vi "NI ELVISmx Set Variable Power Supplies.vi"(0 "Device Name":tag="Dev1", 1 "Stop":bool, 2 "Supply+ (V)":dbl min=0.0 max=12.0, 3 "Supply- (V)":dbl min=-12.0 max=0.0, 5 "error in":errorcluster, 7 "Manual +":bool, 8 "Manual -":bool) -> (16 "Manual +?":bool, 17 "Manual -?":bool, 19 "error out":errorcluster)   [LabVIEW 2014]
doc: "This one shot VI sets the voltage of the positive and negative variable voltage supplies on the ELVIS board. The output can be cleared by running the vi again with the Clear button set to true. If this fails power off the NI Elvis Board.\n\nPaul K Dixon\nPhysics 350\nCSUSB Physics"
uses:
  nilvaiu.dll
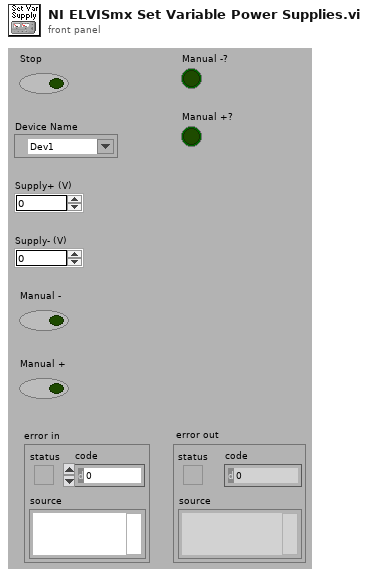
[diagram p1: front panel]
types:
  T1 = typedef "ctl_ProductCategory.ctl" = u16
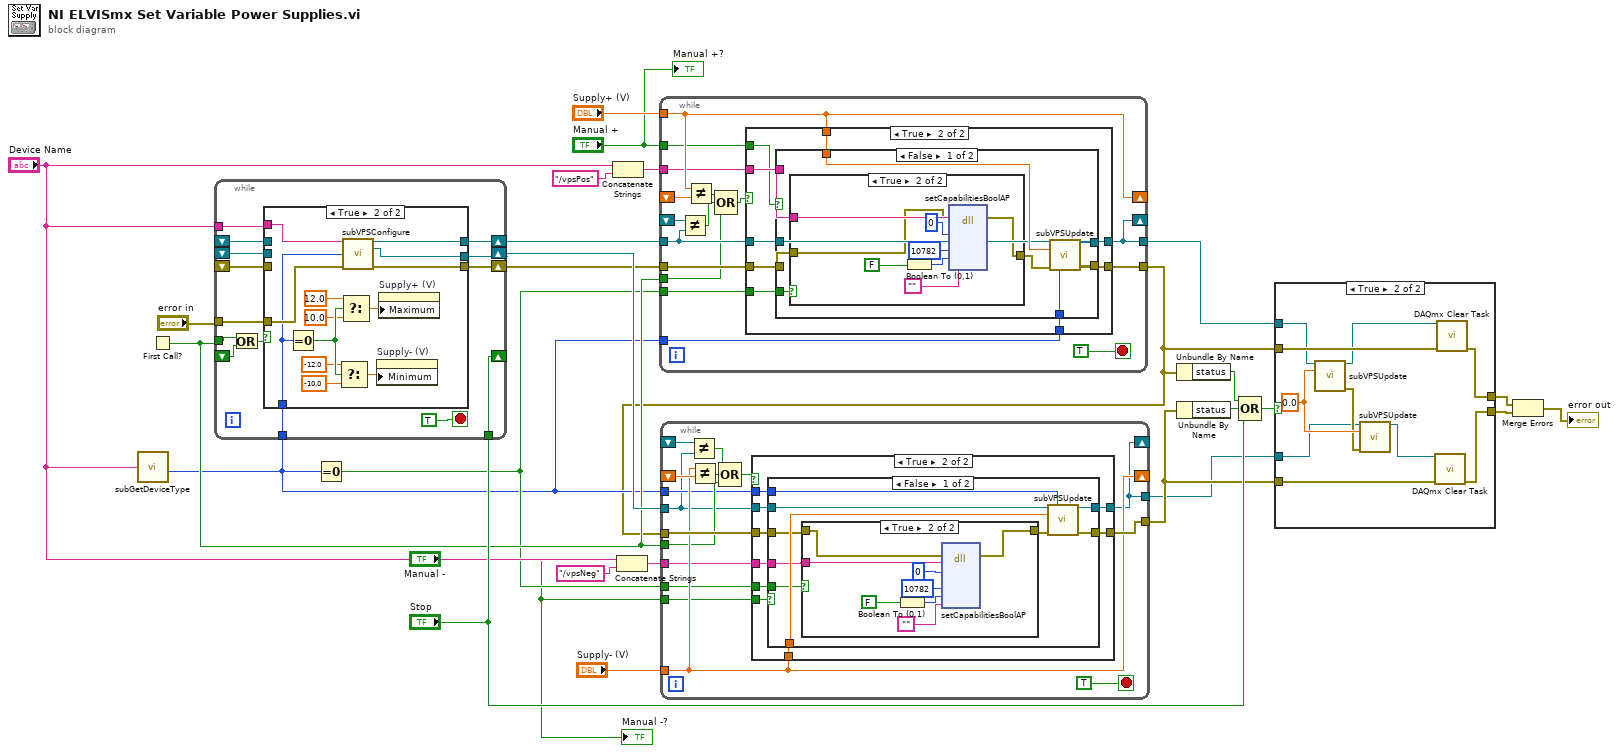
[diagram p0: block diagram]
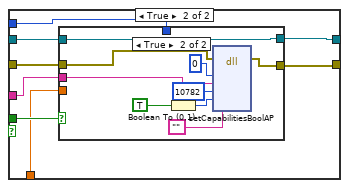
[diagram p4: hidden frame]
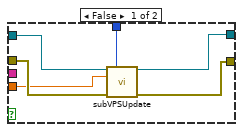
[diagram p5: hidden frame]
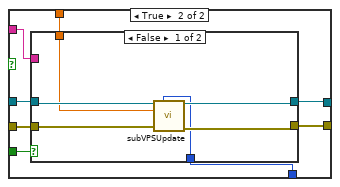
[diagram p8: hidden frame]
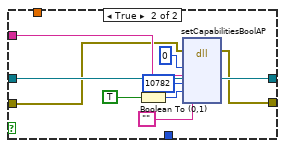
[diagram p9: hidden frame]
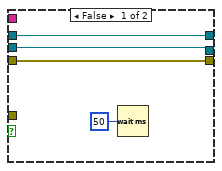
[diagram p11: hidden frame]
diagram:
  n1 = call <vilib>:"subGetDeviceType.vi"("DAQmx Device Name"="Device Name") -> ("Product Category"=w5:T1)  [unwired: 4 out]
  n2 = First Call?() -> (First Call?: T/F=w12:bool)
  n3 = while {
    tunnel: "error in" -> [w41]
    tunnel: w12 -> [w40]
    tunnel: "Device Name" -> [w38]
    tunnel: "Stop" -> [w36]
    shift-right: [w36] -> _
    shift-left: _ -> [w35]
    shift-right: [w34] -> w2
    shift-left: _ -> [w33]
    shift-right: [w32] -> w18
    shift-left: _ -> [w30]
    shift-right: [w31] -> w17
    shift-left: _ -> [w29]
    tunnel: w5 -> [w28]
    stop <- TRUE stop-if-true
    n4 = Or(x=w40, y=w35) -> (x .or. y?=w37:bool)
    n5 = case shown="True" w37 {
      tunnel: [w45 w57] -> w34
      tunnel: w41 -> [_ w58]
      tunnel: w38 -> [_ w46]
      tunnel: w33 -> [w45 _]
      tunnel: [w44 w56] -> w32
      tunnel: [w43 w55] -> w31
      tunnel: w30 -> [w44 _]
      tunnel: w29 -> [w43 _]
      tunnel: w28 -> [_ w52]
      frame False {
        n6 = Wait (ms)(milliseconds to wait=u32 50) -> ()  [unwired: 1 out]
      }
      frame True {
        n7 = Equal To 0?(x=w52) -> (x = 0?=w51:bool)
        n8 = Select(t=-12.0, s=w51, f=-10.0) -> (s? t:f=w53:dbl)
        n9 = Select(t=12.0, s=w51, f=10.0) -> (s? t:f=w54:dbl)
        n10 = call <vilib>:"subVPSConfigure.vi"("Device Name"=w46, "Device Type"=w52, "error in"=w58) -> ("Supply+ task"=w56:refnum<k21>, "Supply- task"=w55:refnum<k21>, "error out"=w57:errorcluster)  [unwired: 10 out]
        n11 = property on="Supply- (V)" class="DigNum (strict)"("Minimum"=w53) -> ()  [unwired: 2 in, 2 out]
        n12 = property on="Supply+ (V)" class="DigNum (strict)"("Maximum"=w54) -> ()  [unwired: 2 in, 2 out]
      }
    }
  }
  n13 = Equal To 0?(x=w5) -> (x = 0?=w6:bool)
  n14 = Concatenate Strings("Device Name", "/vpsPos" ("string")) -> (w9:string)
  n15 = Concatenate Strings("Device Name", "/vpsNeg" ("string")) -> (w8:string)
  n16 = while {
    tunnel: [w74] -> w1
    tunnel: "Supply+ (V)" -> [w69]
    tunnel: w18 -> [w62]
    tunnel: w2 -> [w73]
    tunnel: [w64] -> w13
    shift-right: [w69] -> _
    shift-left: _ -> [w70]
    tunnel: w12 -> [w61]
    tunnel: w9 -> [w67]
    tunnel: w6 -> [w66]
    tunnel: w5 -> [w65]
    shift-right: [w64] -> _
    shift-left: _ -> [w63]
    tunnel: "Manual +" -> [w59]
    stop <- TRUE stop-if-true
    n17 = Not Equal?(x=w63, y=w62) -> (x != y?=w60:bool)
    n18 = Not Equal?(x=w69, y=w70) -> (x != y?=w71:bool)
    n19 = Compound Arithmetic op=OR(w71, w60, w61) -> (w68:bool)
    n20 = case shown="True" w68 {
      tunnel: [w75 w85] -> w74
      tunnel: w69 -> [_ w84]
      tunnel: w62 -> [w76 w83]
      tunnel: w73 -> [w75 w82]
      tunnel: [w76 w81] -> w64
      tunnel: w67 -> [_ w80]
      tunnel: w66 -> [_ w79]
      tunnel: w65 -> [_ w78]
      tunnel: w59 -> [_ w77]
      frame False {
      }
      frame True {
        n21 = case "Manual +" shown="False" w77 {
          tunnel: [w94 w109] -> w85
          tunnel: w84 -> [w93 w105]
          tunnel: w83 -> [w92 w107]
          tunnel: w82 -> [w89 w110]
          tunnel: [w91 w106] -> w81
          tunnel: w80 -> [w90 w111]
          tunnel: w79 -> [w87 w108]
          tunnel: w78 -> [w86 w104]
          frame False {
            n22 = case shown="True" w87 {
              tunnel: w90 -> [_ w98]
              tunnel: w89 -> [w95 w97]
              tunnel: [w95 w96] -> w88
              frame False {
              }
              frame True {
                n23 = Boolean To (0,1)(Boolean=FALSE ("AO.ManualControl.Enable")) -> (0, 1=w100:i16)
                n24 = dll-call lib="nilvaiu.dll" fn="setCapabilitiesBoolAP"(error in=w97, "taskID"=u32 0, "activeProperty"=w98, "attributeID"=10782, "paramValue"=w100, "extendedErrorInfoHdlPtr"="" ("Empty String Constant")) -> (error out=w96:errorcluster)  [unwired: 5 in, 4 out]
              }
            }
            n25 = call <vilib>:"subVPSUpdate.vi"("task ID"=w92, "Device Type"=w86, "Target Voltage"=w93, "error in"=w88) -> ("task out"=w91:refnum<k21>, "error out"=w94:errorcluster)  [unwired: 1 in, 9 out]
          }
          frame True {
            n26 = case shown="False" w108 {
              tunnel: w111 -> [_ w121]
              tunnel: w110 -> [w116 w118]
              tunnel: [w115 w119] -> w109
              tunnel: w107 -> [w117 w126]
              tunnel: [w114 w126] -> w106
              tunnel: w105 -> [w113 _]
              tunnel: w104 -> [w112 _]
              frame False {
                n27 = call <vilib>:"subVPSUpdate.vi"("task ID"=w117, "Device Type"=w112, "Target Voltage"=w113, "error in"=w116) -> ("task out"=w114:refnum<k21>, "error out"=w115:errorcluster)  [unwired: 1 in, 9 out]
              }
              frame True {
                n28 = Boolean To (0,1)(Boolean=TRUE ("AO.ManualControl.Enable")) -> (0, 1=w122:i16)
                n29 = dll-call lib="nilvaiu.dll" fn="setCapabilitiesBoolAP"(error in=w118, "taskID"=u32 0, "activeProperty"=w121, "attributeID"=10782, "paramValue"=w122, "extendedErrorInfoHdlPtr"="" ("Empty String Constant")) -> (error out=w119:errorcluster)  [unwired: 5 in, 4 out]
              }
            }
          }
        }
      }
    }
  }
  n30 = while {
    tunnel: w1 -> [w142]
    tunnel: w17 -> [w129]
    tunnel: "Supply- (V)" -> [w136]
    tunnel: [w141] -> w15
    tunnel: [w131] -> w14
    shift-right: [w136] -> _
    shift-left: _ -> [w137]
    tunnel: w12 -> [w135]
    tunnel: w8 -> [w134]
    tunnel: w6 -> [w133]
    tunnel: w5 -> [w132]
    shift-right: [w131] -> _
    shift-left: _ -> [w130]
    tunnel: "Manual -" -> [w127]
    stop <- TRUE stop-if-true
    n31 = Not Equal?(x=w130, y=w129) -> (x != y?=w128:bool)
    n32 = Not Equal?(x=w136, y=w137) -> (x != y?=w139:bool)
    n33 = Compound Arithmetic op=OR(w128, w139, w135) -> (w138:bool)
    n34 = case shown="True" w138 {
      tunnel: w142 -> [w143 w153]
      tunnel: w129 -> [w144 w152]
      tunnel: w136 -> [_ w151]
      tunnel: [w143 w150] -> w141
      tunnel: [w144 w149] -> w131
      tunnel: w134 -> [_ w148]
      tunnel: w133 -> [_ w147]
      tunnel: w132 -> [_ w146]
      tunnel: w127 -> [_ w145]
      frame False {
      }
      frame True {
        n35 = case "Manual -" shown="False" w145 {
          tunnel: w153 -> [w157 w177]
          tunnel: w152 -> [w162 w175]
          tunnel: w151 -> [w161 w173]
          tunnel: [w160 w178] -> w150
          tunnel: [w159 w174] -> w149
          tunnel: w148 -> [w158 w179]
          tunnel: w147 -> [w155 w176]
          tunnel: w146 -> [w154 w172]
          frame False {
            n36 = case shown="True" w155 {
              tunnel: w158 -> [_ w165]
              tunnel: w157 -> [w163 w166]
              tunnel: [w163 w164] -> w156
              frame False {
              }
              frame True {
                n37 = Boolean To (0,1)(Boolean=FALSE ("AO.ManualControl.Enable")) -> (0, 1=w168:i16)
                n38 = dll-call lib="nilvaiu.dll" fn="setCapabilitiesBoolAP"(error in=w166, "taskID"=u32 0, "activeProperty"=w165, "attributeID"=10782, "paramValue"=w168, "extendedErrorInfoHdlPtr"="" ("Empty String Constant")) -> (error out=w164:errorcluster)  [unwired: 5 in, 4 out]
              }
            }
            n39 = call <vilib>:"subVPSUpdate.vi"("task ID"=w162, "Device Type"=w154, "Target Voltage"=w161, "error in"=w156) -> ("task out"=w159:refnum<k21>, "error out"=w160:errorcluster)  [unwired: 1 in, 9 out]
          }
          frame True {
            n40 = case shown="True" w176 {
              tunnel: w179 -> [_ w188]
              tunnel: [w183 w186] -> w178
              tunnel: w177 -> [w182 w187]
              tunnel: w175 -> [w185 w194]
              tunnel: [w184 w194] -> w174
              tunnel: w173 -> [w181 _]
              tunnel: w172 -> [w180 _]
              frame False {
                n41 = call <vilib>:"subVPSUpdate.vi"("task ID"=w185, "Device Type"=w180, "Target Voltage"=w181, "error in"=w182) -> ("task out"=w184:refnum<k21>, "error out"=w183:errorcluster)  [unwired: 1 in, 9 out]
              }
              frame True {
                n42 = Boolean To (0,1)(Boolean=TRUE ("AO.ManualControl.Enable")) -> (0, 1=w190:i16)
                n43 = dll-call lib="nilvaiu.dll" fn="setCapabilitiesBoolAP"(error in=w187, "taskID"=u32 0, "activeProperty"=w188, "attributeID"=10782, "paramValue"=w190, "extendedErrorInfoHdlPtr"="" ("Empty String Constant")) -> (error out=w186:errorcluster)  [unwired: 5 in, 4 out]
              }
            }
          }
        }
      }
    }
  }
  n44 = Unbundle By Name(w1) -> ("status"=w23:bool)
  n45 = Unbundle By Name(w15) -> ("status"=w21:bool)
  n46 = Compound Arithmetic op=OR(w23, w21, "Stop") -> (w22:bool)
  n47 = case shown="True" w22 {
    tunnel: w1 -> [w196 w203]
    tunnel: w15 -> [w195 w199]
    tunnel: [w196 w206] -> w25
    tunnel: [w195 w205] -> w24
    tunnel: w14 -> [_ w198]
    tunnel: w13 -> [_ w201]
    frame False {
    }
    frame True {
      w204 = 0.0 ("Target Voltage")
      n48 = call <vilib>:"subVPSUpdate.vi"("task ID"=w201, "Target Voltage"=w204) -> ("task out"=w200:refnum<k21>, "error out"=w202:errorcluster)  [unwired: 3 in, 9 out]
      n49 = call <vilib>:"subVPSUpdate.vi"("task ID"=w198, "Target Voltage"=w204, "error in"=w202) -> ("task out"=w197:refnum<k21>)  [unwired: 2 in, 10 out]
      n50 = call <vilib>:"DAQmx Clear Task.vi"("task in"=w197, "error in"=w199) -> ("error out"=w205:errorcluster)  [unwired: 13 out]
      n51 = call <vilib>:"DAQmx Clear Task.vi"("task in"=w200, "error in"=w203) -> ("error out"=w206:errorcluster)  [unwired: 13 out]
    }
  }
  n52 = Merge Errors(w25, w24) -> (→"error out":errorcluster)
  "Manual -?" <- "Manual -"
  "Manual +?" <- "Manual +"
